vi "Interactive Test.vi"() -> ()   [LabVIEW 2013, in "HadCon.lvlib"]
uses:
  <instrlib>/HadCon/HadCon.lvlib
panel:
  out "Response":string
  in  "Command":string
  out "Error Out":errorcluster
  in  "VISA resource name":refnum<visa-resource-name>
  out "Instrument Firmware Revision":string
  out "Instrument Driver Revision":string
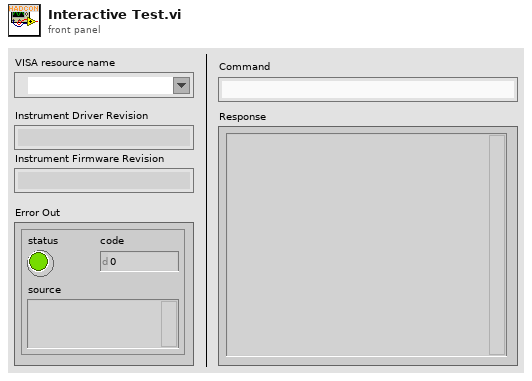
[diagram p1: front panel]
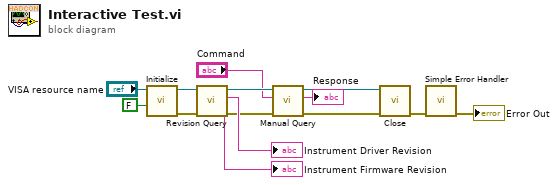
[diagram p0: block diagram]
diagram:
  n1 = call <instrlib>:"Initialize.vi"("Reset (True)"=FALSE, "VISA resource name"="VISA resource name") -> ("error out"=w13:errorcluster, "VISA resource name out"=w14:refnum<visa-resource-name>)  [unwired: 8 in]
  n2 = call <instrlib>:"Revision Query.vi"("error in (no error)"=w13, "VISA resource name"=w14) -> ("error out"=w6:errorcluster, "Instrument Firmware Revision"=→"Instrument Firmware Revision":string, "Instrument Driver Revision"=→"Instrument Driver Revision":string, "VISA resource name out"=w7:refnum<visa-resource-name>)  [unwired: 6 in]
  n3 = call <instrlib>:"Manual Query.vi"("error in (no error)"=w6, "Command"="Command", "VISA resource name"=w7) -> ("error out"=w4:errorcluster, "Response"=→"Response":string, "VISA resource name out"=w5:refnum<visa-resource-name>)  [unwired: 6 in]
  n4 = call <instrlib>:"Close.vi"("error in (no error)"=w4, "VISA resource name"=w5) -> ("error out"=w10:errorcluster)  [unwired: 9 in]
  n5 = call <vilib>:"Simple Error Handler.vi"("error in (no error)"=w10) -> ("error out"=→"Error Out":errorcluster)  [unwired: 4 in, 4 out]
